vi "PixyCam_SetServos.vi"(4 "error in (no error)":errorcluster, 5 "Tilt Servo Position":u16 max=1000, 6 "Pan Servo Position":u16 max=1000, 7 "PixyCamDevRef":T1) -> (0 "error out":errorcluster, 3 "PixyCamDevRef Out":T1)   [LabVIEW 2016, in "PixyCam_LabVIEW.lvlib"]
uses:
  PixyCam_LabVIEW.lvlib
  Private/PixyCam_DevRef.ctl
  Private/PixyCam_SPI_DevRef.ctl
  <vilib>/Rock Robotics/WPI/SPI/WPI_SPIDevRef.ctl
  <vilib>/Rock Robotics/SystemInterfaces/spilib/spi_bus.ctl
  Private/PixyCam_CommMode.ctl
  Private/PixyCam_SerialByteConstants.ctl
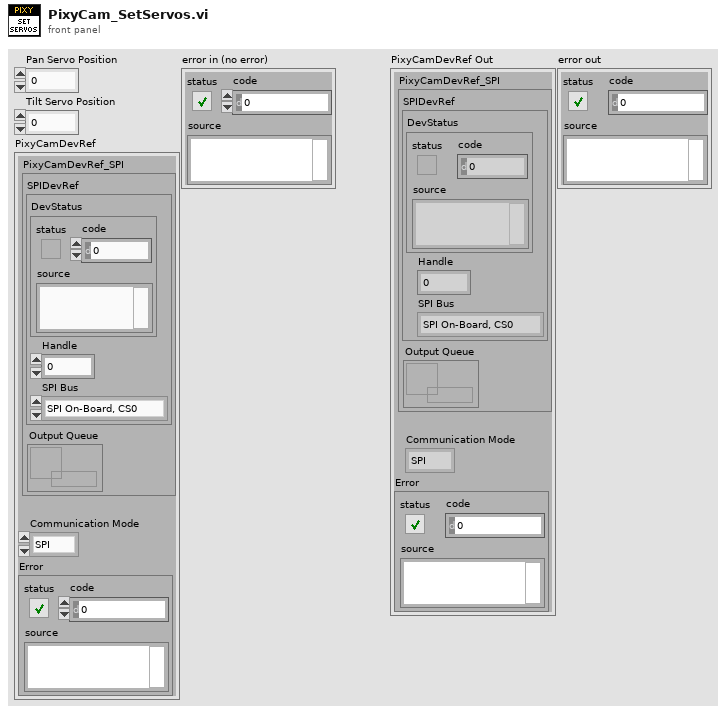
[diagram p1: front panel]
types:
  T1 = typedef "PixyCam_LabVIEW.lvlib/PixyCam_DevRef.ctl" = cluster{"PixyCamDevRef_SPI":T2, "Communication Mode":T5, "Error":errorcluster}
  T2 = typedef "PixyCam_LabVIEW.lvlib/PixyCam_SPI_DevRef.ctl" = cluster{"SPIDevRef":T3, "Output Queue":refnum<queue>}
  T3 = typedef "WPI_SPIDevRef.ctl" = cluster{"DevStatus":errorcluster, "Handle":i32, "SPI Bus":T4}
  T4 = typedef "spi_bus.ctl" = enum16{"SPI On-Board, CS0", "SPI On-Board, CS1", "SPI On-Board, CS2", "SPI On-Board, CS3", "SPI MXP", "Invalid"}
  T5 = typedef "PixyCam_LabVIEW.lvlib/PixyCam_CommMode.ctl" = enum16{"SPI", "I2C", "UART", "Analog", "Digital"}
  T6 = typedef "PixyCam_LabVIEW.lvlib/PixyCam_SerialByteConstants.ctl" = u8
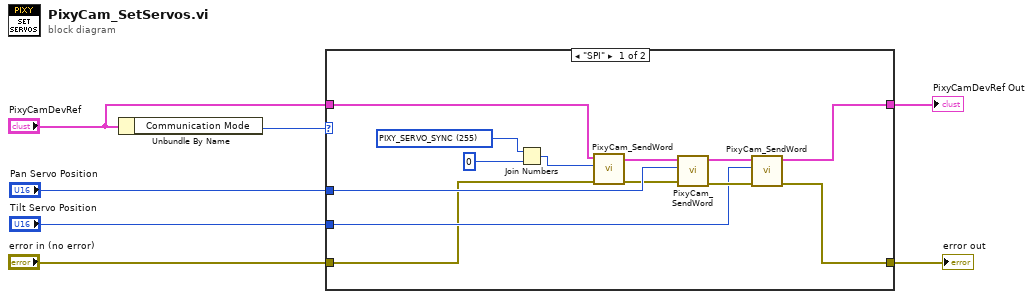
[diagram p0: block diagram]
diagram:
  n1 = Unbundle By Name("PixyCamDevRef") -> ("Communication Mode"=w7:T5)
  n2 = case shown="\"SPI\"" w7 {
    tunnel: "PixyCamDevRef" -> [w12 w22]
    tunnel: "error in (no error)" -> [w14 w21]
    tunnel: "Pan Servo Position" -> [w20 _]
    tunnel: "Tilt Servo Position" -> [w17 _]
    tunnel: [w16 w22] -> w2
    tunnel: [w15 w21] -> w1
    frame "SPI" {
      w11 = T6 255 items=["PIXY_SYNC_BYTE"=90, "PIXY_SYNC_BYTE_DATA"=91, "PIXY_SERVO_SYNC"=255, "PIXY_CAM_BRIGHTNESS_SYNC"=254, "PIXY_CAM_LED_SYNC"=253] ("SyncByte")
      n3 = Join Numbers(hi=w11, lo=u8 0 ("timeout in ms (-1)")) -> ((hi.lo)=w9:u16)
      n4 = call "PixyCam_SendWord.vi"("error in"=w14, "WriteWord"=w9, "PixyCamDevRef"=w12) -> ("error out"=w8:errorcluster, "PixyCamDevRef Out"=w13:T1)  [unwired: 3 in]
      n5 = call "PixyCam_SendWord.vi"("error in"=w8, "WriteWord"=w20, "PixyCamDevRef"=w13) -> ("error out"=w19:errorcluster, "PixyCamDevRef Out"=w18:T1)  [unwired: 3 in]
      n6 = call "PixyCam_SendWord.vi"("error in"=w19, "WriteWord"=w17, "PixyCamDevRef"=w18) -> ("error out"=w15:errorcluster, "PixyCamDevRef Out"=w16:T1)  [unwired: 3 in]
    }
    frame Default {
    }
  }
  "PixyCamDevRef Out" <- w2
  "error out" <- w1
